vi "Exemple_Metrics_Silhouette_Score.vi"() -> ()   [LabVIEW 2020]
uses:
  Objet/3 - Model selection and evaluation/3.3 - Metrics and scoring/silhouette_score/Silhouette_Score.vi
panel:
  out "Score":string
  out "error out":errorcluster caption="sortie d'erreur"
  in  "error in (no error)":errorcluster caption="entrée d'erreur (pas d'erreur)"
  in  "silhouette_score":T1={"metric"="euclidean", "sample_size"="None", "random_state"=-1} {"random_state" min=-1}
  in  "labels":string[][](array[string])=[["0"], ["1"], ["1"]]
  in  "X":string[][](array[string])=[["0", "1"], ["2", "3"], ["4", "5"]]
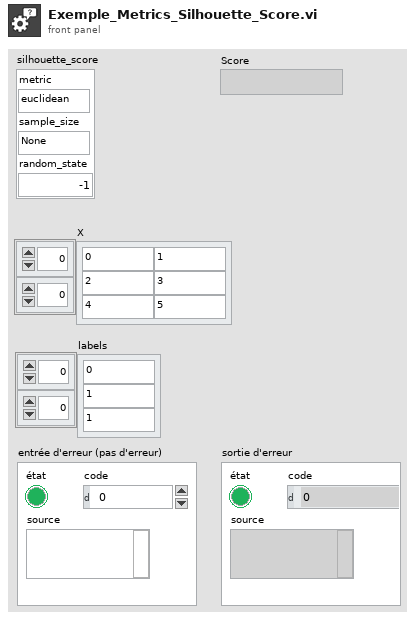
[diagram p1: front panel]
types:
  T1 = cluster{"metric":string, "sample_size":string, "random_state":i32}
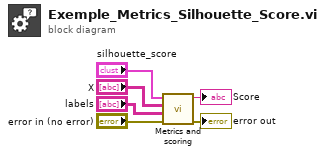
[diagram p0: block diagram]
diagram:
  n1 = call-poly "Metrics and scoring.vi"("error in (no error)"="error in (no error)", "labels"="labels", "X"="X", "silhouette_score"="silhouette_score") -> ("error out"=→"error out":errorcluster, "Score"=→"Score":string)  [unwired: 6 in]
